vi "sent by autofocus QM.vi"(8 "error in (no error)":errorcluster, 10 "ProceedMessage":refnum<class "ProceedMessage.lvclass">, 11 "Autofocus in":refnum<class "Autofocus.lvclass">) -> (0 "error out":errorcluster, 1 "sent by autofocus?":bool, 2 "ProceedMessage 2":refnum<class "ProceedMessage.lvclass">, 3 "Autofocus out":refnum<class "Autofocus.lvclass">)   [LabVIEW 2012, in "Autofocus.lvclass"]
uses:
  Autofocus.lvclass
  <vilib>/Distrio/Murmex/ProceedMessage/ProceedMessage.lvclass
  <vilib>/Distrio/Murmex/Murmex/Murmex.lvclass
  <vilib>/Distrio/Murmex/Message/Message.lvclass
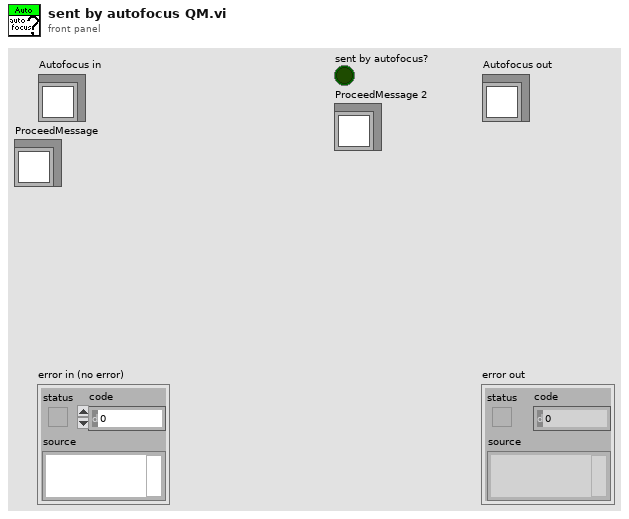
[diagram p1: front panel]
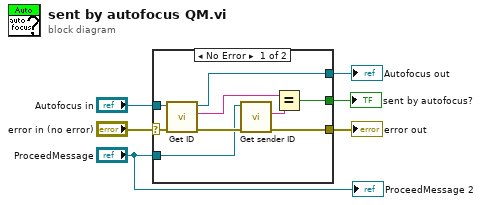
[diagram p0: block diagram]
diagram:
  n1 = case shown="No Error" "error in (no error)" {
    selector: "error in (no error)" -> [w13 w17]
    tunnel: [w10 w17] -> w5
    tunnel: [w14 w16] -> w3
    tunnel: "Autofocus in" -> [w15 w16]
    tunnel: "ProceedMessage" -> [w9 _]
    tunnel: [w8 _] -> w1
    frame No Error {
      n2 = call <vilib>:"Get ID.vi"("error in (no error)"=w13, "Murmex in"=w15) -> ("error out"=w11:errorcluster, "component id"=w12:string, "Murmex out"=w14:refnum<class "Autofocus.lvclass">)  [unwired: 7 in]
      n3 = call <vilib>:"Get sender ID.vi"("error in (no error)"=w11, "Message in"=w9) -> ("error out"=w10:errorcluster, "sender"=w7:string)  [unwired: 7 in, 1 out]
      n4 = Equal?(x=w12, y=w7) -> (x = y?=w8:bool)
    }
    frame Error {
    }
  }
  "error out" <- w5
  "Autofocus out" <- w3
  "sent by autofocus?" <- w1
  "ProceedMessage 2" <- "ProceedMessage"
